vi "ROTATION SELECT.vi"(9 "ROTATION CONTROL":enum16{"POV hat ", "TWIST axis"}(ring), 10 "POVs in":i16[](array[numeric]), 11 "TWIST in":dbl) -> (3 "Jr":dbl)   [LabVIEW 2023]
panel:
  in  "Spin\nMIN":dbl=0.4 format="%#_13g"
  in  "Spin\nMAX":dbl=1.0 format="%#_13g"
  in  "Max dx/dt\nTWIST":dbl=10.0
  in  "Max dx/dt\nPOV":dbl=10.0
  in  "deadband\nTWIST":dbl=0.1 format="%#_13g"
  in  "Reset":bool
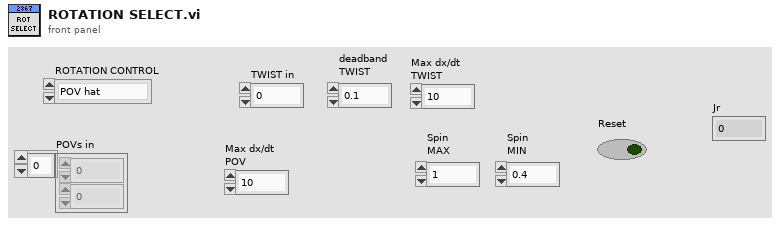
[diagram p1: front panel]
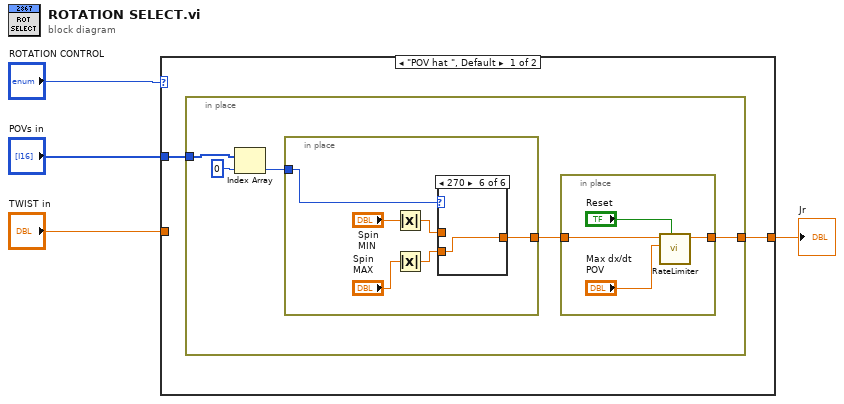
[diagram p0: block diagram]
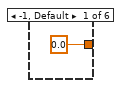
[diagram p2: hidden frame]
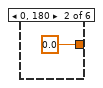
[diagram p3: hidden frame]
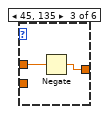
[diagram p4: hidden frame]
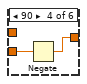
[diagram p5: hidden frame]
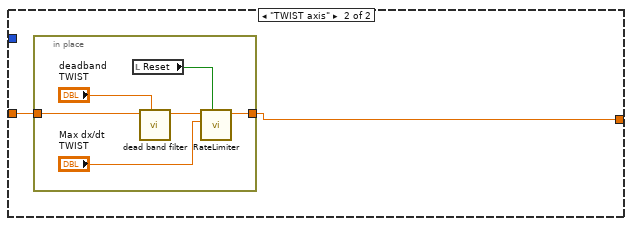
[diagram p7: hidden frame]
diagram:
  n1 = case shown="\"POV hat \", Default" "ROTATION CONTROL" {
    tunnel: [w6 w31] -> w4
    tunnel: "TWIST in" -> [_ w30]
    tunnel: "POVs in" -> [w5 _]
    frame "POV hat ", Default {
      n2 = in-place {
        in-place-border: [w10] -> w6
        in-place-border: w5 -> [w7]
        n3 = Index Array(array=w7, index=0) -> (element=w9:i16)
        n4 = in-place {
          in-place-border: w9 -> [w15]
          in-place-border: [w14] -> w8
          n5 = Absolute Value(x="Spin\nMIN") -> (abs(x)=w12:dbl)
          n6 = Absolute Value(x="Spin\nMAX") -> (abs(x)=w13:dbl)
          n7 = case shown="270" w15 {
            tunnel: [0.0 ("Output") 0.0 ("Output") w20 w22 w24 w25] -> w14
            tunnel: w12 -> [_ _ w21 _ w24 _]
            tunnel: w13 -> [_ _ _ w23 _ w25]
            frame -1, Default {
            }
            frame 0, 180 {
            }
            frame 45, 135 {
              n8 = Negate(x=w21) -> (-x=w20:dbl)
            }
            frame 90 {
              n9 = Negate(x=w23) -> (-x=w22:dbl)
            }
            frame 225, 315 {
            }
            frame 270 {
            }
          }
        }
        n10 = in-place {
          in-place-border: [w27] -> w10
          in-place-border: w8 -> [w26]
          n11 = call "RateLimiter.vi"("Reset"="Reset", "Max dx/dt"="Max dx/dt\nPOV", "Input"=w26) -> ("Output"=w27:dbl)  [unwired: 8 in]
        }
      }
    }
    frame "TWIST axis" {
      n12 = in-place {
        in-place-border: [w35] -> w31
        in-place-border: w30 -> [w33]
        n13 = local read "Reset"() -> (w32:bool)
        n14 = call "dead band filter.vi"("deadband"="deadband\nTWIST", "input"=w33) -> ("output"=w34:dbl)  [unwired: 9 in]
        n15 = call "RateLimiter.vi"("Reset"=w32, "Max dx/dt"="Max dx/dt\nTWIST", "Input"=w34) -> ("Output"=w35:dbl)  [unwired: 8 in]
      }
    }
  }
  "Jr" <- w4
